vi "Raster Scan Init.vi"(6 "Resolution (nm/pixel)":dbl[unit], 7 "Start":dbl[unit], 8 "Bins per scan":dbl, 9 "Bin width (nm)":dbl[unit], 10 "Bin width (pixels)":dbl, 11 "End":dbl[unit]) -> (1 "Empty Data Array":cluster{dbl[unit], dbl[]}[](array[cluster]), 2 "Spec First Position":dbl[unit], 3 "Number of snapshots":dbl)   [LabVIEW 2017, in "Synapse CCD.lvclass"]
uses:
  Synapse CCD.lvclass
panel:
  out "Number of data points in scan":dbl
  in  "Total Pixel Count":dbl=1024.0
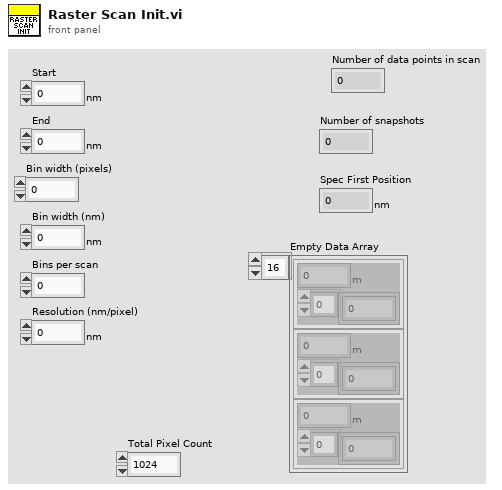
[diagram p1: front panel]
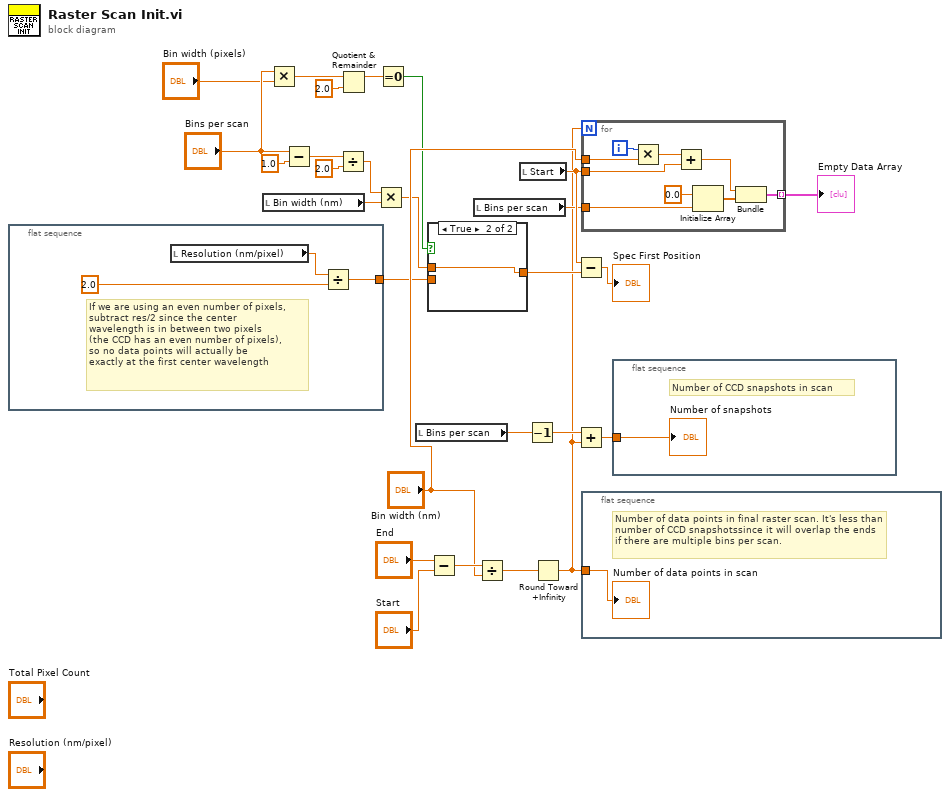
[diagram p0: block diagram]
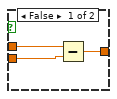
[diagram p2: hidden frame]
diagram:
  n1 = flat-sequence {
    tunnel: [w28] -> w7
    frame #0 {
      # "If we are using an even number of pixels, \nsubtract res/2 since the center\nwavelength is in between two pixels\n(the CCD has an even number of pixels), \nso no data points will actually be \nexactly at the first center wavelength"
      n2 = local read "Resolution (nm/pixel)"() -> (w29:dbl[unit])
      n3 = Divide(x=w29, y=2.0) -> (x/y=w28:dbl[unit])
    }
  }
  n4 = local read "Bin width (nm)"() -> (w16:dbl[unit])
  n5 = Multiply(x="Bins per scan", y="Bin width (pixels)") -> (x*y=w4:dbl)
  n6 = Subtract(x="Bins per scan", y=1.0) -> (x-y=w25:dbl)
  n7 = Divide(x=w25, y=2.0) -> (x/y=w23:dbl)
  n8 = Quotient & Remainder(x=w4, y=2.0) -> (x-y*floor(x/y)=w9:dbl)  [unwired: 1 out]
  n9 = Multiply(x=w23, y=w16) -> (x*y=w11:dbl[unit])
  n10 = Equal To 0?(x=w9) -> (x = 0?=w8:bool)
  n11 = local read "Bins per scan"() -> (w3:dbl)
  n12 = case shown="True" w8 {
    tunnel: w11 -> [w33 w34]
    tunnel: [w31 w34] -> w10
    tunnel: w7 -> [w32 _]
    frame False {
      n13 = Subtract(x=w33, y=w32) -> (x-y=w31:dbl[unit])
    }
    frame True {
    }
  }
  n14 = Subtract(x="End", y="Start") -> (x-y=w17:dbl[unit])
  n15 = local read "Bins per scan"() -> (w14:dbl)
  n16 = Divide(x=w17, y="Bin width (nm)") -> (x/y=w27:dbl)
  n17 = local read "Start"() -> (w18:dbl[unit])
  n18 = Decrement(x=w3) -> (x-1=w2:dbl)
  n19 = Round Toward +Infinity(x=w27) -> (ceil(x): smallest int >= x=w1:dbl)
  n20 = Subtract(x=w18, y=w10) -> (x-y=→"Spec First Position":dbl[unit])
  n21 = Add(x=w2, y=w1) -> (x+y=w19:dbl)
  n22 = for {
    N: w1 -> [_]
    tunnel: "Bin width (nm)" -> [w42]
    tunnel: w18 -> [w40]
    tunnel: [w37] -> w22 mode=indexing
    tunnel: w14 -> [w36]
    i -> [w43]
    n23 = Multiply(x=w43, y=w42) -> (x*y=w41:dbl[unit])
    n24 = Add(x=w41, y=w40) -> (x+y=w35:dbl[unit])
    n25 = Initialize Array(0.0 ("element"), w36) -> (w38:dbl[])
    n26 = Bundle(w35, w38) -> (w37:cluster{dbl[unit], dbl[]})  [unwired: 1 in]
  }
  "Empty Data Array" <- w22
  n27 = flat-sequence {
    tunnel: w1 -> [w44]
    frame #0 {
      # "Number of data points in final raster scan. It's less than number of CCD snapshotssince it will overlap the ends if there are multiple bins per scan."
      "Number of data points in scan" <- w44
    }
  }
  n28 = flat-sequence {
    tunnel: w19 -> [w45]
    frame #0 {
      # "Number of CCD snapshots in scan"
      "Number of snapshots" <- w45
    }
  }
